vi "ui.vi"() -> ()   [LabVIEW 2017]
panel:
  out "波形图":dbl[](graph)
  in  "布尔":bool
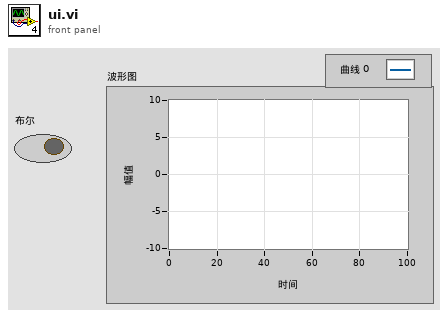
[diagram p1: front panel]
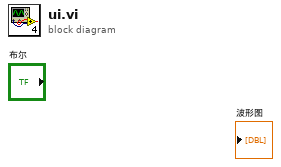
[diagram p0: block diagram]
diagram:
